vi "Initialize.vi"(8 "error in (no error)":errorcluster, 9 "Reset (True)":bool=TRUE, 10 "ID Query (True)":bool=TRUE, 11 "VISA resource name":refnum<visa-resource-name>) -> (0 "error out":errorcluster, 3 "VISA resource name out":refnum<visa-resource-name>)   [LabVIEW 2024, in "Keithley 2200 Series.lvlib"]
doc: "Establishes communication with the power supply by finding the USB address.Call this VI before calling other instrument driver VIs. Generally, you need to call the power supply Initialize VI only once at the beginning of an application.The values in bracket are default values."
uses:
  Keithley 2200 Series.lvlib
panel:
  # "(c) Copyright 2012 Keithley Instruments Inc  ALL RIGHTS RESERVED."
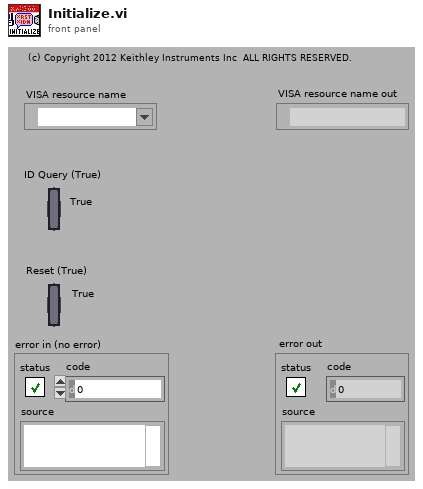
[diagram p1: front panel]
types:
  T1 = cluster{"status":bool, "code":i32, "VI Name":string}
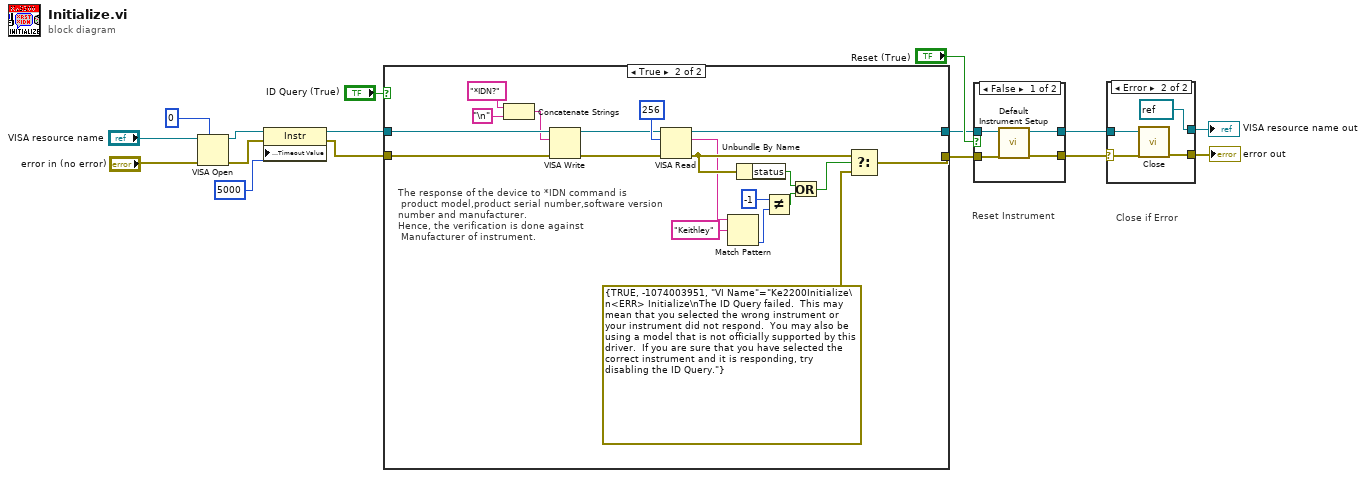
[diagram p0: block diagram]
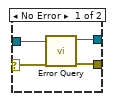
[diagram p2: hidden frame]
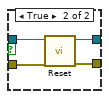
[diagram p3: hidden frame]
diagram:
  # "Close if Error"
  # "Reset Instrument"
  n1 = VISA Open(timeout (0)=u32 0 ("VISA Open timeout (0)"), error in (no error)="error in (no error)", VISA resource name="VISA resource name") -> (VISA resource name=w7:refnum<visa-resource-name>, error out=w6:errorcluster)  [unwired: 2 out]
  n2 = property on="Property Node" class="Instr"(reference=w7, error in=w6, "General Settings:Timeout Value"=u32 5000 ("Timeout (10000)")) -> (reference out=w3:refnum<visa-resource-name>, error out=w2:errorcluster)
  n3 = case shown="True" "ID Query (True)" {
    tunnel: [w18 w34] -> w13
    tunnel: [w17 w27] -> w12
    tunnel: w2 -> [w17 w33]
    tunnel: w3 -> [w18 w32]
    frame False {
    }
    frame True {
      # "The response of the device to *IDN command is\n product model,product serial number,software version\nnumber and manufacturer.\nHence, the verification is done against\n Manufacturer of instrument."
      n4 = Concatenate Strings("*IDN?" ("write buffer"), "\n" ("End of Line Constant")) -> (w30:string)
      n5 = VISA Write(VISA resource name=w32, write buffer=w30, error in (no error)=w33) -> (VISA resource name out=w36:refnum<visa-resource-name>, error out=w35:errorcluster)  [unwired: 1 out]
      n6 = VISA Read(VISA resource name=w36, byte count=u32 256, error in (no error)=w35) -> (VISA resource name out=w34:refnum<visa-resource-name>, read buffer=w19:string, error out=w26:errorcluster)  [unwired: 1 out]
      n7 = Match Pattern(string=w19, regular expression="Keithley") -> (offset past match=w24:i32)  [unwired: 4 out]
      n8 = Unbundle By Name(w26) -> ("status"=w22:bool)
      n9 = Not Equal?(x=-1, y=w24) -> (x != y?=w21:bool)
      n10 = Or(x=w22, y=w21) -> (x .or. y?=w20:bool)
      n11 = Select(t=w26, s=w20, f=cluster{bool, i32, "VI Name":string} {TRUE, -1074003951, "VI Name"="Ke2200Initialize\n<ERR> Initialize\nThe ID Query failed.  This may mean that you selected the wrong instrument or your instrument did not respond.  You may also be using a model that is not officially supported by this driver.  If you are sure that you have selected the correct instrument and it is responding, try disabling the ID Query."}) -> (s? t:f=w27:T1)
    }
  }
  n12 = case shown="False" "Reset (True)" {
    tunnel: w13 -> [w41 w43]
    tunnel: w12 -> [w40 w45]
    tunnel: [w39 w42] -> w11
    tunnel: [w38 w44] -> w10
    frame False {
      n13 = call "Default Instrument Setup.vi"("error in (no error)"=w40, "VISA resource name"=w41) -> ("error out"=w38:errorcluster, "VISA resource name out"=w39:refnum<visa-resource-name>)  [unwired: 8 out]
    }
    frame True {
      n14 = call "Reset.vi"("error in (no error)"=w45, "VISA resource name"=w43) -> ("error out"=w44:errorcluster, "VISA resource name out"=w42:refnum<visa-resource-name>)  [unwired: 8 out]
    }
  }
  n15 = case shown="Error" w10 {
    selector: w10 -> [w49 w53]
    tunnel: [w48 refnum<visa-resource-name> refnum ("VISA resource name Out")] -> w14
    tunnel: w11 -> [w46 w51]
    tunnel: [w47 w52] -> w9
    frame No Error {
      n16 = call "Error Query.vi"("error in (no error)"=w49, "VISA resource name"=w46) -> ("error out"=w47:errorcluster, "VISA resource name out"=w48:refnum<visa-resource-name>)  [unwired: 8 out]
    }
    frame Error {
      n17 = call "Close.vi"("error in (no error)"=w53, "VISA resource name"=w51) -> ("error out"=w52:errorcluster)  [unwired: 9 out]
    }
  }
  "error out" <- w9
  "VISA resource name out" <- w14
